vi "tdms image file ref.vi"(10 "command":enum16{"set", "get"}(ring)=enum."get", 11 "tdms file ref":refnum<k34>) -> (3 "tdms file ref":refnum<k34>)   [LabVIEW 2020]
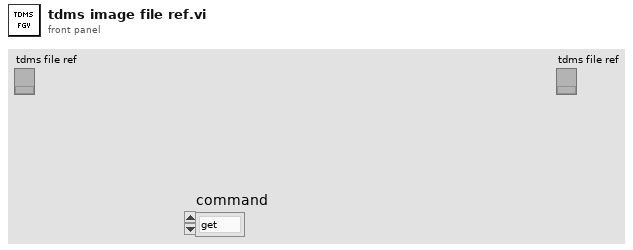
[diagram p1: front panel]
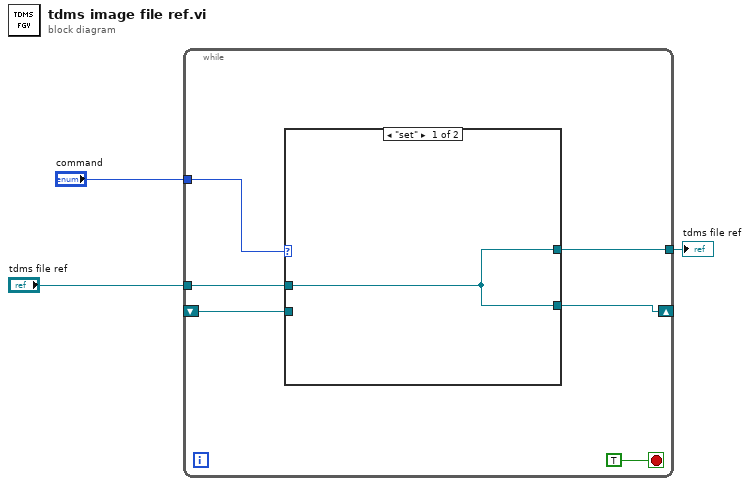
[diagram p0: block diagram]
diagram:
  n1 = while {
    shift-right: [w5] -> _
    shift-left: _ -> [w7]
    tunnel: "command" -> [w8]
    tunnel: [w6] -> w2
    tunnel: "tdms file ref" -> [w4]
    stop <- TRUE stop-if-true
    n2 = case shown="\"set\"" w8 {
      tunnel: [w10 w11] -> w6
      tunnel: w7 -> [_ w11]
      tunnel: [w10 w11] -> w5
      tunnel: w4 -> [w10 _]
      frame "set" {
      }
      frame "get", Default {
      }
    }
  }
  "tdms file ref" <- w2
